vi "Shift Function.vi"(0 "N":dbl, 1 "Vshift":dbl, 2 "Template":dbl[](graph)) -> (5 "Waveform Graph":dbl[](graph))   [LabVIEW 2016]
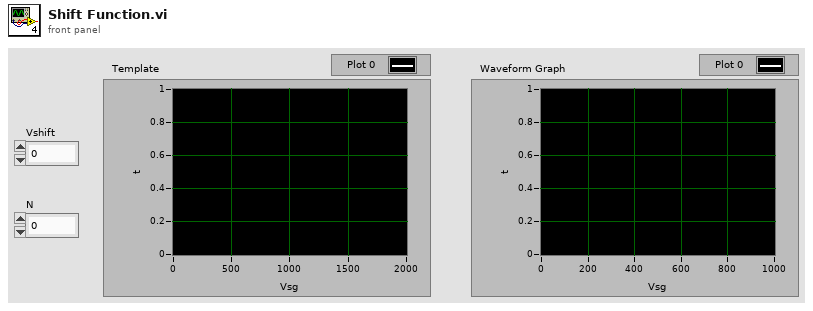
[diagram p1: front panel]
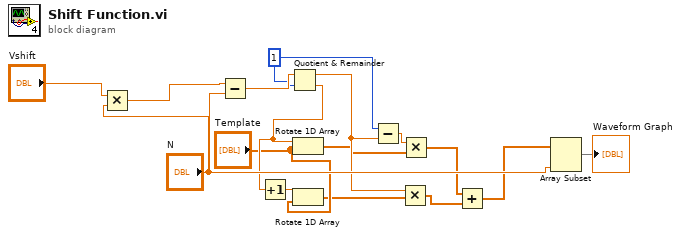
[diagram p0: block diagram]
diagram:
  w8 = 1
  n1 = Multiply(x="Vshift", y="N") -> (x*y=w13:dbl)
  n2 = Subtract(x=w13, y="N") -> (x-y=w12:dbl)
  n3 = Quotient & Remainder(x=w12, y=w8) -> (x-y*floor(x/y)=w5:dbl, floor(x/y)=w10:dbl)
  n4 = Increment(x=w10) -> (x+1=w11:dbl)
  n5 = Rotate 1D Array(1:"Template", 2:w10) -> (0:w1:dbl[])
  n6 = Rotate 1D Array(1:"Template", 2:w11) -> (0:w6:dbl[])
  n7 = Subtract(x=w8, y=w5) -> (x-y=w7:dbl)
  n8 = Multiply(x=w5, y=w6) -> (x*y=w4:dbl[])
  n9 = Multiply(x=w7, y=w1) -> (x*y=w3:dbl[])
  n10 = Add(x=w3, y=w4) -> (x+y=w2:dbl[])
  n11 = Array Subset(array=w2, length="N") -> (→"Waveform Graph":dbl[])  [unwired: 1 in]
